vi "Hello World.vi"   [LabVIEW 2017]
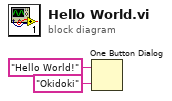
[diagram p0: block diagram]
diagram:
  n1 = One Button Dialog(message="Hello World!", button name ("OK")="Okidoki") -> ()  [unwired: 1 out]
